vi "reflectiesensor_signalen  (SubVI).vi"() -> ()   [LabVIEW 2019]
uses:
  <vilib>/myRIO/Instrument Drivers/Onboard IO/AI/AI.lvlib
panel:
  out "de afgeleid":dbl[](array[numeric])
  out "de vorige gemeten waarde":dbl[](array[numeric])
  out "de gemeten waarde":dbl[](array[numeric])
  out "error out":errorcluster
  in  "error in (no error)":errorcluster
  in  "namen van analoge inputs  in 2":tag[](array[tag])
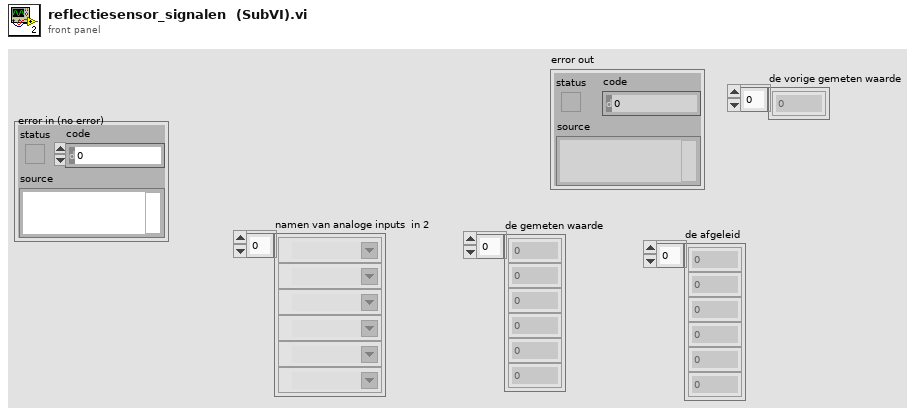
[diagram p1: front panel]
types:
  T1 = typedef "AI.lvlib/AI Reference.ctl" = cluster{"myRIO Reference":T2, "AI Channels List":T6, "AI Scaling Constants List":T8}
  T2 = typedef "myRIO Generic Hardware Reference.ctl" = cluster{"myRIO Model":T3, "myRIO Hardware Reference":T4}
  T3 = typedef "Hardware Version Enum.ctl" = enum16{"Unknown", "myRIO-1900", "myRIO-1950", "roboRIO", "NI ELVIS RIO CM", "ELVIS III"}
  T4 = typedef "myRIO v1.0 Reference.ctl" = cluster{"Generic FPGA Reference":T5, "Allow multiple opens":bool}
  T5 = typedef "Generic FPGA Reference.ctl" = refnum<k20>
  T6 = typedef "AI Channels List.ctl" = T7[]
  T7 = typedef "AI Channels Enum.ctl" = enum16{"Not Connected", "AudioIn/Left", "AudioIn/Right", "C/AI0", "C/AI1", "A/AI0", "A/AI1", "A/AI2", "A/AI3", "A/AI4", "A/AI5", "A/AI6", "A/AI7", "B/AI0", "B/AI1", "B/AI2", "B/AI3", "B/AI4", "B/AI5", "B/AI6", "B/AI7", "AI/AI0", "AI/AI1", "AI/AI2", "AI/AI3", "A/AI0 (DIFF)", "A/AI1 (DIFF)", "A/AI2 (DIFF)", "A/AI3 (DIFF)", "B/AI0 (DIFF)", "B/AI1 (DIFF)", "B/AI2 (DIFF)", "B/AI3 (DIFF)"}
  T8 = typedef "Analog Scaling Constants List.ctl" = T9[]
  T9 = typedef "Analog Scaling Constants.ctl" = cluster{"LSB Weight (Volts)":dbl, "Offset (Volts)":dbl, "Signed?":bool}
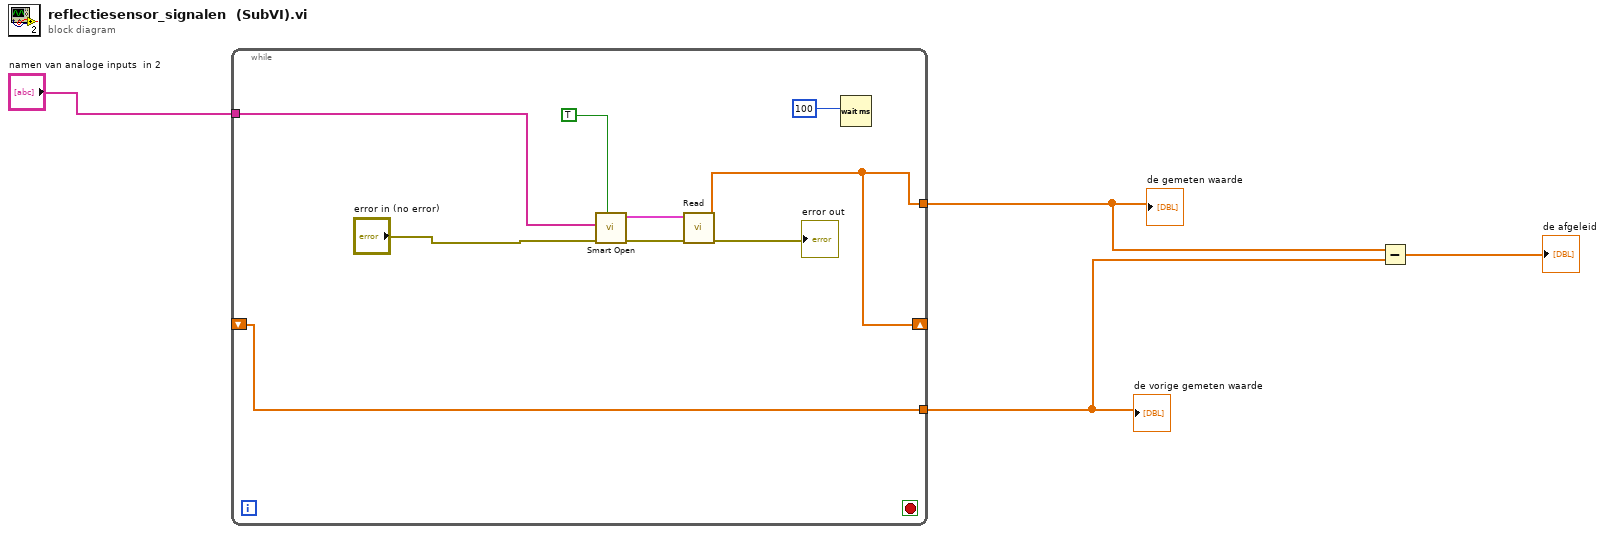
[diagram p0: block diagram]
diagram:
  n1 = while {
    tunnel: [w9] -> w3
    shift-right: [w9] -> _
    shift-left: _ -> [w8]
    tunnel: [w8] -> w2
    tunnel: "namen van analoge inputs  in 2" -> [w6]
    stop <- _ stop-if-true
    n2 = call <vilib>:"Smart Open.vi"("Allow multiple opens?"=TRUE, "error in (no error)"="error in (no error)", "Channel Names"=w6) -> ("error out"=w12:errorcluster, "AI Ref Out"=w13:T1)  [unwired: 7 in]
    n3 = call <vilib>:"Read.vi"("error in (no error)"=w12, "AI Ref In"=w13) -> ("error out"=→"error out":errorcluster, "Values"=w9:dbl[])  [unwired: 7 in, 1 out]
    n4 = Wait (ms)(milliseconds to wait=100) -> ()  [unwired: 1 out]
  }
  "de gemeten waarde" <- w3
  "de vorige gemeten waarde" <- w2
  n5 = Subtract(x=w3, y=w2) -> (x-y=→"de afgeleid":dbl[])
